vi "Get Resource Type.vi"(4 "AnalogIn in":refnum<class "AI.lvclass">) -> (7 "Resource Type":string)   [LabVIEW 2020, in "CTI.lvlib" / "AI.lvclass"]
uses:
  AI.lvclass
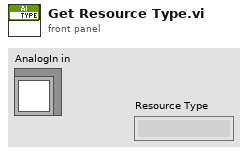
[diagram p1: front panel]
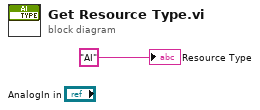
[diagram p0: block diagram]
diagram:
  "Resource Type" <- "AI" ("Resource Type")
